vi "Load Enabled Instrument List.vi"(8 "error in":errorcluster, 11 "Manual UI in":refnum<class "Manual UI.lvclass">) -> (0 "error out":errorcluster, 3 "Manual UI out":refnum<class "Manual UI.lvclass">)   [LabVIEW 2023, in "Manual UI.lvlib" / "Manual UI.lvclass"]
doc: "This routine loads the config.ini file, filters out devices that are not instruments, or not enabled, and returns a list of enabled instruments to launch. \n\nThis is a pre-instrument launch directive, meant to be called immediately before launching instruments in case the user changes the configuration at run time."
uses:
  Project/Manual UI.lvclass
  Project/Manual UI.lvclass/Manual UI.ctl
  Accessors/Read Config.vi
  builds/Tools/Config.lvlibp/Accessors/Read Device List.vi
  builds/Tools/Config.lvlibp/Accessors/Write Device.vi
  builds/Tools/Config.lvlibp/Config.lvclass
  builds/Instruments/Instruments.lvlibp/Library/Instruments.lvclass
  builds/Engine/Engine.lvlibp/Project/Engine.lvclass
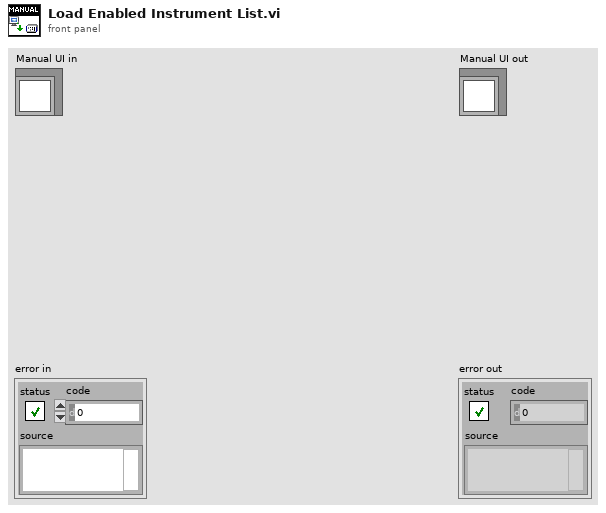
[diagram p1: front panel]
types:
  T1 = cluster{"String":string, "Instrument":refnum<class "Instruments.lvclass">, i32}
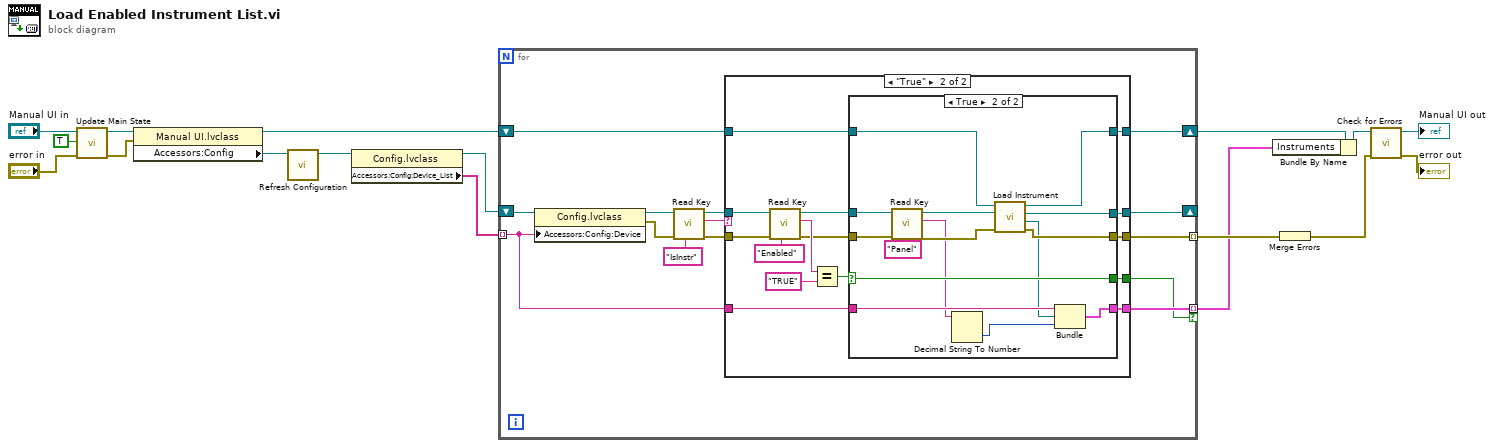
[diagram p0: block diagram]
diagram:
  n1 = call "Update Main State.vi"("error in"="error in", "Loading"=TRUE, "Manual UI in"="Manual UI in") -> ("error out"=w2:errorcluster, "Manual UI out"=w3:refnum<class "Manual UI.lvclass">)  [unwired: 7 in]
  n2 = property class="Manual UI.lvclass"(reference=w3, error in=w2) -> (reference out=w8:refnum<class "Manual UI.lvclass">, "Accessors:Config"=w10:refnum<class "Config.lvclass">)  [unwired: 1 out]
  n3 = call "Refresh Configuration.vi"("Config in"=w10) -> ("Config out"=w9:refnum<class "Config.lvclass">)  [unwired: 9 in, 1 out]
  n4 = property class="Config.lvclass"(reference=w9) -> (reference out=w16:refnum<class "Config.lvclass">, "Accessors:Config:Device_List"=w17:string[])  [unwired: 1 in, 1 out]
  n5 = for {
    tunnel: w17 -> [w22] mode=indexing
    shift-right: [w25] -> _
    shift-left: w16 -> [w31]
    tunnel: [w23] -> w15 mode=indexing
    tunnel: [w21] -> w6 mode=indexing if=w20
    shift-right: [w18] -> w7
    shift-left: w8 -> [w19]
    n6 = property class="Config.lvclass"(reference=w31, "Accessors:Config:Device"=w22) -> (reference out=w30:refnum<class "Config.lvclass">, error out=w29:errorcluster)  [unwired: 1 in]
    n7 = call "Read Key.vi"("Key Name"="IsInstr", "error in"=w29, "Config in"=w30) -> ("error out"=w24:errorcluster, "Key Value"=w27:string, "Config out"=w26:refnum<class "Config.lvclass">)  [unwired: 6 in]
    n8 = case shown="\"True\"" w27 {
      tunnel: w26 -> [w34 w48]
      tunnel: [w34 w40] -> w25
      tunnel: w24 -> [w33 w49]
      tunnel: [w33 w39] -> w23
      tunnel: [_ w43] -> w20
      tunnel: w22 -> [_ w36]
      tunnel: [_ w35] -> w21
      tunnel: w19 -> [w32 w38]
      tunnel: [w32 w37] -> w18
      frame "False", Default {
      }
      frame "True" {
        n9 = call "Read Key.vi"("Key Name"="Enabled", "error in"=w49, "Config in"=w48) -> ("error out"=w41:errorcluster, "Key Value"=w46:string, "Config out"=w42:refnum<class "Config.lvclass">)  [unwired: 6 in]
        n10 = Equal?(x=w46, y="TRUE") -> (x = y?=w44:bool)
        n11 = case shown="True" w44 {
          selector: w44 -> [w50 w68]
          tunnel: [w50 w68] -> w43
          tunnel: w42 -> [w52 w59]
          tunnel: w41 -> [w51 w60]
          tunnel: [w52 w67] -> w40
          tunnel: [w51 w66] -> w39
          tunnel: w38 -> [w53 w65]
          tunnel: [w53 w64] -> w37
          tunnel: w36 -> [_ w63]
          tunnel: [_ w61] -> w35
          frame False {
          }
          frame True {
            n12 = call "Read Key.vi"("Key Name"="Panel", "error in"=w60, "Config in"=w59) -> ("error out"=w57:errorcluster, "Key Value"=w55:string, "Config out"=w58:refnum<class "Config.lvclass">)  [unwired: 6 in]
            n13 = Decimal String To Number(string=w55) -> (number=w54:i32)  [unwired: 2 in, 1 out]
            n14 = call "Load Instrument.vi"("error in"=w57, "Config in"=w58, "Manual UI in"=w65) -> ("error out"=w66:errorcluster, "Instrument"=w62:refnum<class "Instruments.lvclass">, "Config out"=w67:refnum<class "Config.lvclass">, "Manual UI out"=w64:refnum<class "Manual UI.lvclass">)  [unwired: 5 in]
            n15 = Bundle("String"=w63, "Instrument"=w62, w54) -> (w61:T1)  [unwired: 1 in]
          }
        }
      }
    }
  }
  n16 = Bundle By Name(cluster=w7, "Instruments"=w6) -> (w13:refnum<class "Manual UI.lvclass">)
  n17 = Merge Errors(w15) -> (w11:errorcluster)
  n18 = call "Check for Errors.vi"("error in"=w11, "Engine in"=w13) -> ("error out"=→"error out":errorcluster, "Engine out"=→"Manual UI out":refnum<class "Manual UI.lvclass">)  [unwired: 8 in]
